vi "FPGA_9505_Thruster_PWMGeneratorOnly_NoCurrentFBack.vi"() -> ()   [LabVIEW 2012]
uses:
  <vilib>/LabVIEW Targets/FPGA/cRIO/cRIO-9505/controls.llb/_nicrio_cRIO-9505_DriveStatus.ctl
  <vilib>/Platform/TimedLoop/XDataNode/timing_clust.ctl
  <vilib>/Platform/TimedLoop/XDataNode/nitl_modes.ctl
  <vilib>/Platform/TimedLoop/XDataNode/wakeup.ctl
  <vilib>/LabVIEW Targets/FPGA/cRIO/cRIO-9505/controls.llb/_nicrio_cRIO-9505_DriveDirection.ctl
  <vilib>/rvi/Emulation/niFpgaSctlEmulationRegisterWithScheduler.vi
  <vilib>/rvi/Emulation/niFpgaSctlEmulationScheduler.vi
  <vilib>/rvi/eio/common/nirviEmuTemplateMethod_errors.vi
  <vilib>/rvi/eio/common/nirviEmuTemplatePropertyGet_noerrors.vi
  <vilib>/rvi/Emulation/niFpgaSctlEmulationGlobalWrite.vi
  <vilib>/Platform/TimedLoop/XDataNode/XDataNode.xnode
  <vilib>/eio/EIONode/EIONode.xnode
  <vilib>/eio/EIOMethodNode/EIOMethodNode.xnode
  <vilib>/eio/EIOPropertyNode/EIOPropertyNode.xnode
  <vilib>/rvi/eio/common/nirviEmuTemplatePropertyGet_errors.vi
  <vilib>/rvi/eio/common/nirviEmuTemplatePropertySet_errors.vi
  <vilib>/rvi/eio/common/nirviEmuTemplatePropertySet_noerrors.vi
  <vilib>/Platform/TimedLoop/XDataNode/XDNodeRunTimeDep.lvlib
panel:
  in  "Tab Control":enum32{"Control", "Debugging 1", "Debugging 2"}(tab)
  out "PWM Duty Cycle 1":i16
  in  "Input PWM Loop\nRate (usec) 1":u32=50
  in  "Input PWM 1":i16 caption="Setpoint"
  out "PWM Duty Cycle 2":i16
  in  "Input PWM Loop\nRate (usec) 2":u32=50
  in  "Input PWM 2":i16 caption="Setpoint"
  out "PWM Loop Counter 1":i32(graph)
  out "Sample Current Loop Counter 1":i32(graph)
  out "Current Sense 1":i16(graph)
  in  "Trig AI 1":bool
  out "PWM Duty Cycle 1":i16(graph)
  out "Input PWM Loop Counter 1":i32(graph)
  out "PWM Loop Counter 2":i32(graph)
  out "PWM Duty Cycle 2":i16(graph)
  out "Input PWM Loop Counter 2":i32(graph)
  in  "Trig AI 2":bool
  out "Current Sense 2":i16(graph)
  out "Sample Current Loop Counter 2":i32(graph)
  out "Vsup Present 2":bool
  out "Drive Fault 2":bool
  out "Drive Status 2":T1
  out "Temp Fault 2":bool
  in  "Enable\nDrive 2":bool
  in  "Disable\nDrive 2":bool
  out "Vsup Present 1":bool
  out "Drive Fault 1":bool
  out "Drive Status 1":T1
  out "Temp Fault 1":bool
  in  "Enable\nDrive 1":bool
  in  "Disable\nDrive 1":bool
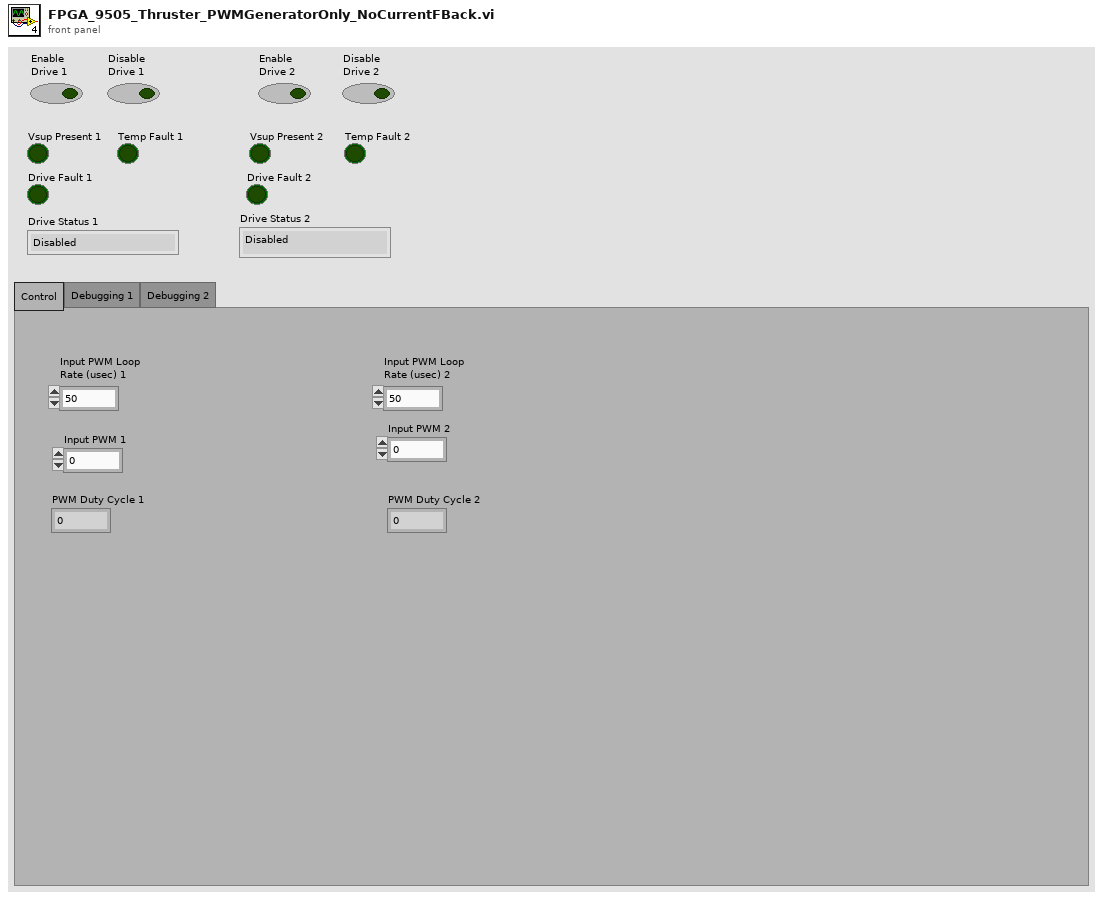
[diagram p1: front panel]
types:
  T1 = typedef "_nicrio_cRIO-9505_DriveStatus.ctl" = enum8{"Enabled", "Disabled", "Disabled by Drive Fault", "Disabled by Temp. Fault", "Disabled by E-Stop", "Unknown"}
  T2 = typedef "XDNodeRunTimeDep.lvlib/timing_clust.ctl" = cluster{"Expected End [f-1]":u64, "Actual End [f-1]":u64, "Finished Late? [f-1]":bool, "Expected End [i-1]":u64, "Actual End [i-1]":u64, "Finished Late? [i-1]":bool, "Expected Start [i]":u64, "Actual Start [i]":u64, "Expected Start [f]":u64, "Actual Start [f]":u64, "Source Name":string, "Structure Name":string, "Period":i64, "Deadline":i64, "Offset":i64, "Start":i64, "Priority":i32, "Timeout":i32, "Mode":T3, "Wakeup Reason":T4, "Error":errorcluster, "Source Type":string, "Secondary Source Type":string, "Global End Time":u64, "Global Start Time":u64, "Frame Duration":u64, "Iteration Duration":u64, "Assigned CPU":i32, "I/O Scan Engine Mode":u32}
  T3 = typedef "XDNodeRunTimeDep.lvlib/nitl_modes.ctl" = enum32{"No Change", "Process missed periods, maintain original phase", "Discard missed periods, maintain original phase", "Process missed periods, ignore original phase", "Discard missed periods, ignore original phase"}
  T4 = typedef "XDNodeRunTimeDep.lvlib/wakeup.ctl" = enum32{"Normal", "Aborted", "Asynchronous wakeup", "Timing source error", "Timed loop error", "Timeout"}
  T5 = typedef "_nicrio_cRIO-9505_DriveDirection.ctl" = enum8{"Clockwise", "Counterclockwise"}
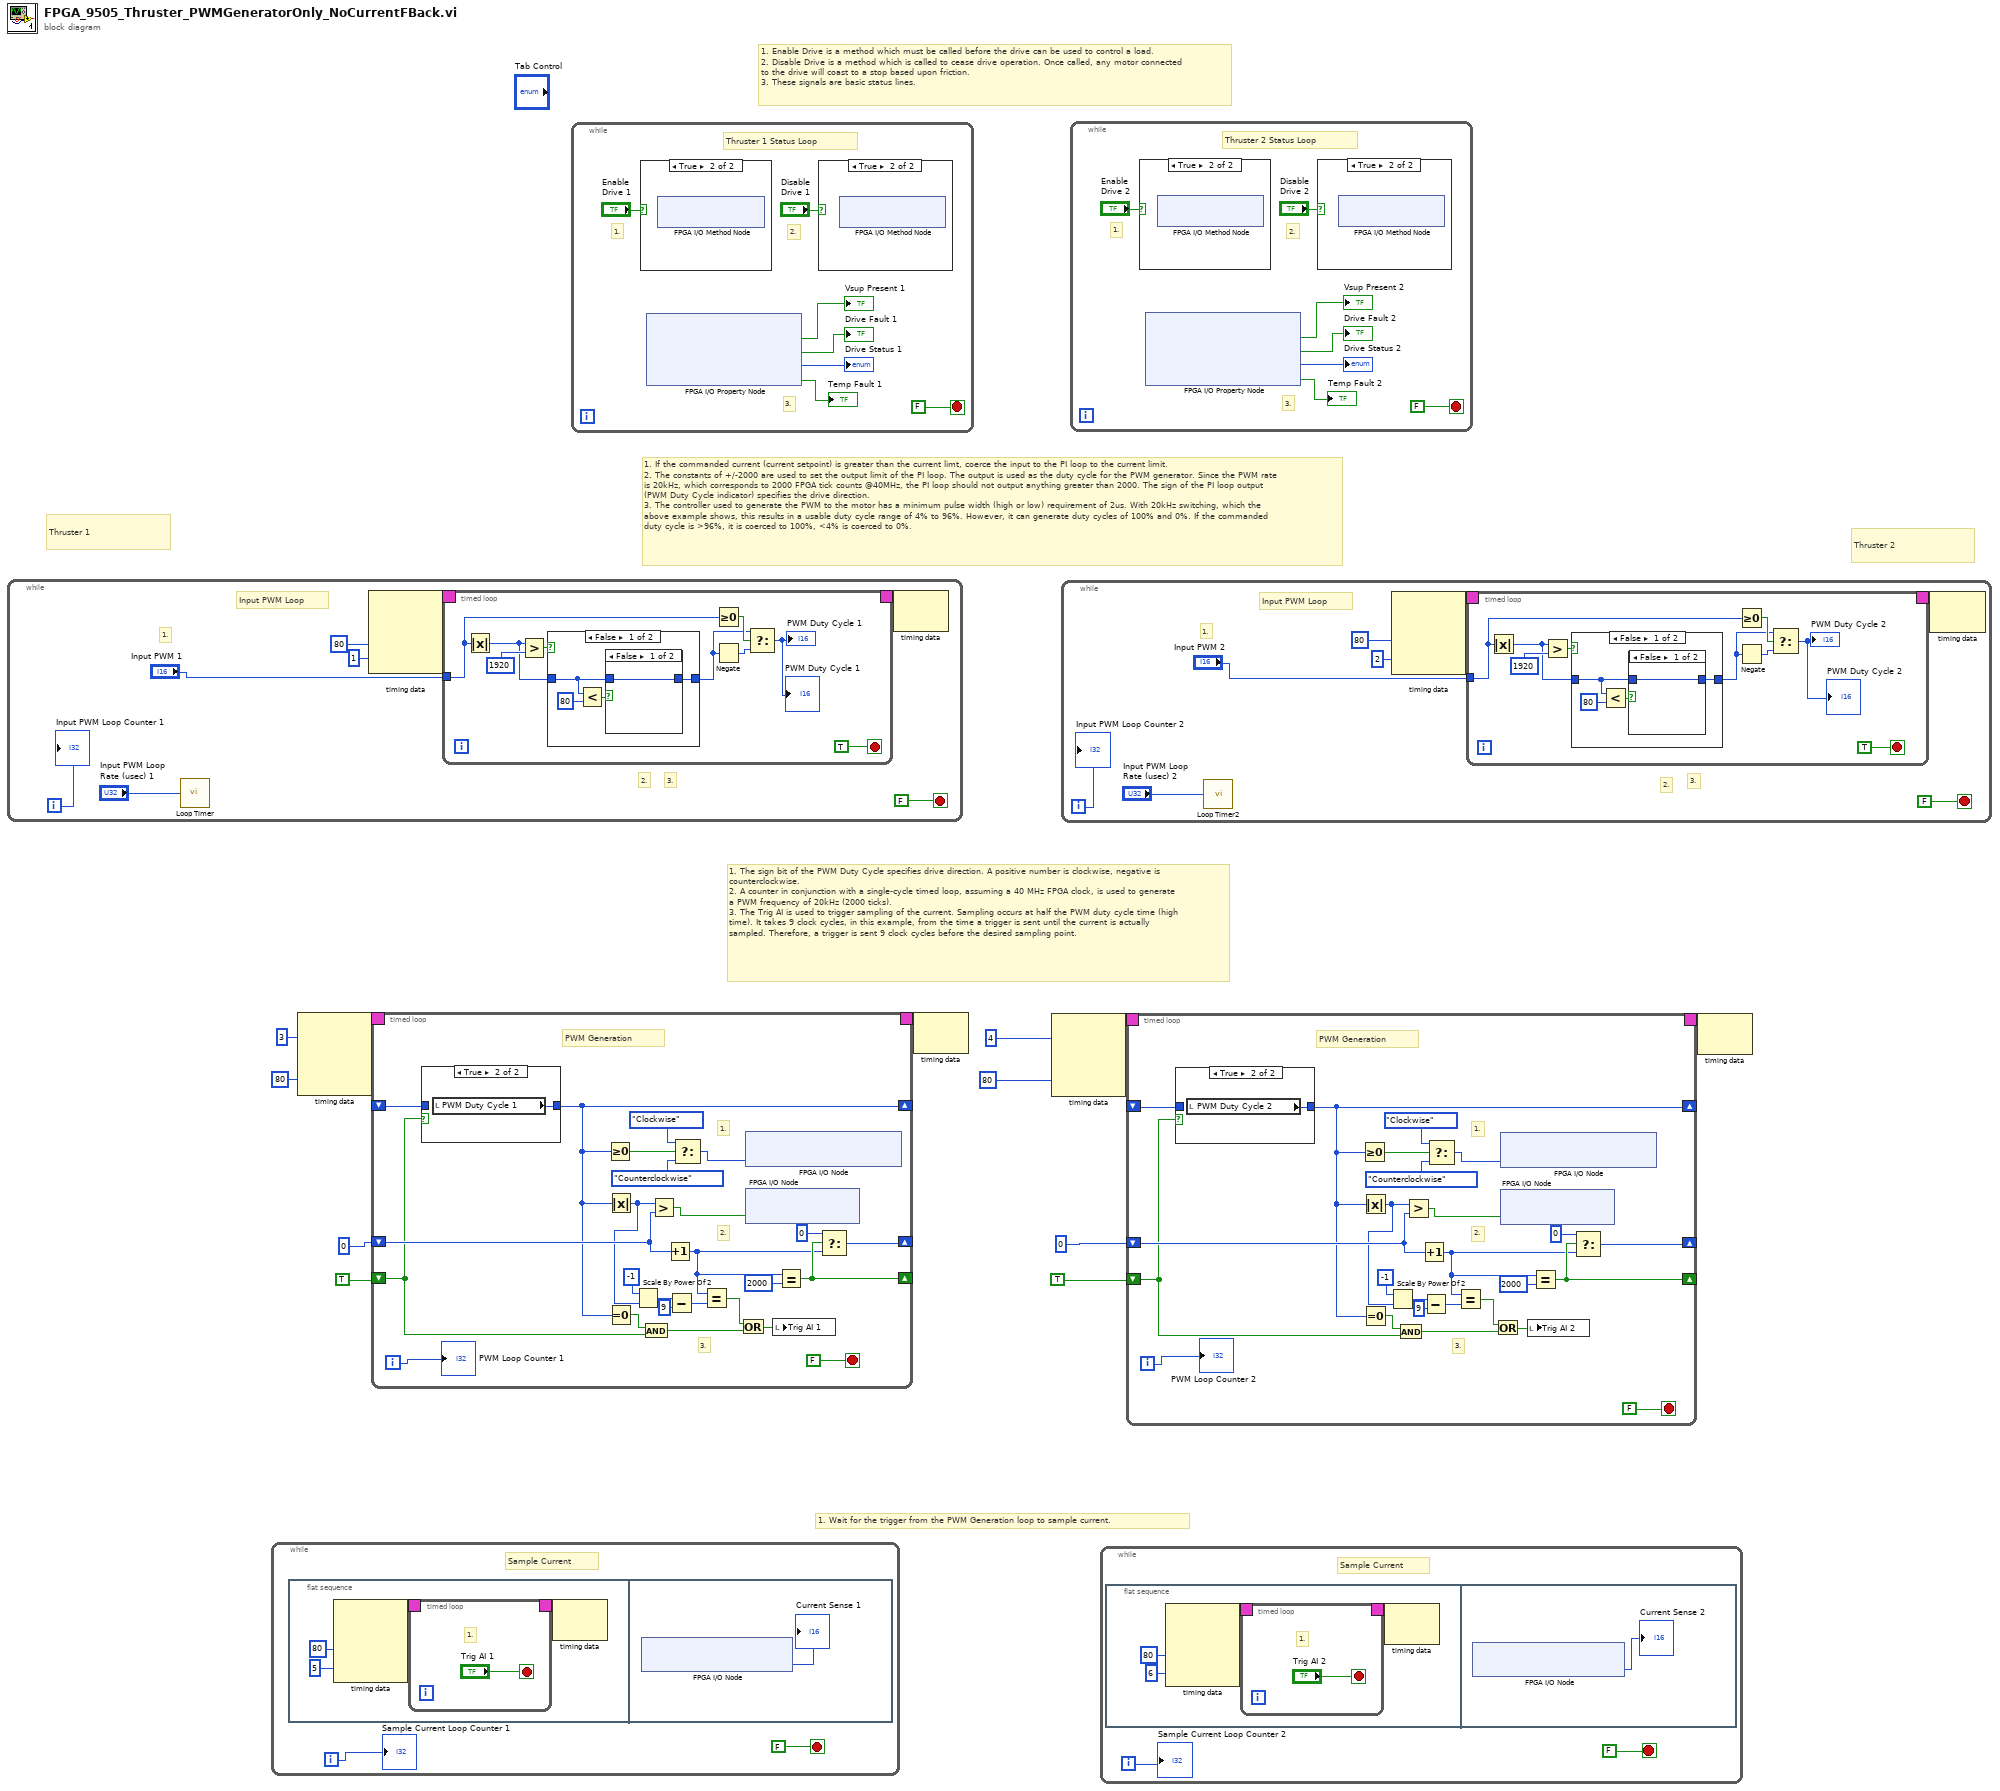
[diagram p0: block diagram]
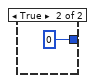
[diagram p4: hidden frame]
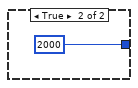
[diagram p5: hidden frame]
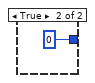
[diagram p6: hidden frame]
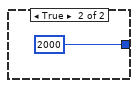
[diagram p7: hidden frame]
diagram:
  # "1. Wait for the trigger from the PWM Generation loop to sample current."
  # "1. The sign bit of the PWM Duty Cycle specifies drive direction. A positive number is clockwise, negative is counterclockwise.\n2. A counter in conjunction with a single-cycle timed loop, assuming a 40 MHz FPGA clock, is used to generate a PWM frequency of 20kHz (2000 ticks).\n3. The Trig AI is used to trigger sampling of the current. Sampling occurs at half the PWM duty cycle time (high time). It takes 9 clock cycles, in this example, from the time a trigger is sent until the current is actually sampled. Therefore, a trigger is sent 9 clock cycles before the desired sampling point."
  # "1. If the commanded current (current setpoint) is greater than the current limt, coerce the input to the PI loop to the current limit.\n2. The constants of +/-2000 are used to set the output limit of the PI loop. The output is used as the duty cycle for the PWM generator. Since the PWM rate is 20kHz, which corresponds to 2000 FPGA tick counts @40MHz, the PI loop should not output anything greater than 2000. The sign of the PI loop output (PWM Duty Cycle indicator) specifies the drive direction.\n3. The controller used to generate the PWM to the motor has a minimum pulse width (high or low) requirement of 2us. With 20kHz switching, which the above example shows, this results in a usable duty cycle range of 4% to 96%. However, it can generate duty cycles of 100% and 0%. If the commanded duty c..."
  # "Thruster 2"
  # "Thruster 1"
  # "1. Enable Drive is a method which must be called before the drive can be used to control a load.\n2. Disable Drive is a method which is called to cease drive operation. Once called, any motor connected to the drive will coast to a stop based upon friction.\n3. These signals are basic status lines."
  n1 = while {
    i -> [w16]
    stop <- FALSE stop-if-true
    # "2."
    # "3."
    # "1."
    # "Input PWM Loop"
    n2 = call "Loop Timer"("Count(uSec)"="Input PWM Loop\nRate (usec) 1") -> ()  [unwired: 1 out]
    n3 = node-c288(80, 1) -> (w19:T2)  [unwired: 2 out]
    n4 = timed-loop {
      timing: w19 -> [_]
      timing-out: [_] -> w18
      tunnel: "Input PWM 1" -> [w23]
      stop <- TRUE stop-if-true
      n5 = Absolute Value(x=w23) -> (abs(x)=w24:i16)
      n6 = Greater?(x=w24, y=i16 1920) -> (0:w26:bool)
      n7 = case shown="False" w26 {
        tunnel: [w32 i16 2000] -> w25
        tunnel: w24 -> [w30 _]
        frame False {
          n8 = Less?(x=w30, y=i16 80) -> (x < y?=w31:bool)
          n9 = case shown="False" w31 {
            tunnel: [w34 i16 0] -> w32
            tunnel: w30 -> [w34 _]
            frame False {
            }
            frame True {
            }
          }
        }
        frame True {
        }
      }
      n10 = Greater Or Equal To 0?(x=w23) -> (x >= 0?=w29:bool)
      n11 = Negate(x=w25) -> (-x=w28:i16)
      n12 = Select(t=w25, s=w29, f=w28) -> (s? t:f=→"PWM Duty Cycle 1" →"PWM Duty Cycle 1":i16)
    }
    n13 = node-c288(w18) -> ()  [unwired: 1 out]
    "Input PWM Loop Counter 1" <- w16
  }
  n14 = while {
    i -> [w44]
    stop <- FALSE stop-if-true
    # "Sample Current"
    n15 = flat-sequence {
      frame #0 {
        n16 = node-c288(80, 5) -> (w49:T2)  [unwired: 2 out]
        n17 = timed-loop {
          timing: w49 -> [_]
          timing-out: [_] -> w48
          stop <- "Trig AI 1" stop-if-true
          # "1."
        }
        n18 = node-c288(w48) -> ()  [unwired: 1 out]
      }
      frame #1 {
        n19 = xnode "FPGA I/O Node"() -> ("Mod2/Current Sense 2"=→"Current Sense 1":i16)  [unwired: 1 in, 1 out]
      }
    }
    "Sample Current Loop Counter 1" <- w44
  }
  n20 = node-c288(3, 80) -> (w12:T2)  [unwired: 2 in]
  n21 = timed-loop {
    timing: w12 -> [_]
    timing-out: [_] -> w11
    shift-right: [w80] -> _
    shift-left: i16 0 -> [w83]
    shift-right: [w79] -> _
    shift-left: TRUE -> [w76]
    shift-right: [w65] -> _
    shift-left: _ -> [w78]
    i -> [w59]
    stop <- FALSE stop-if-true
    # "3."
    # "2."
    # "1."
    # "PWM Generation"
    n22 = case shown="True" w76 {
      tunnel: [w84 w85] -> w65
      tunnel: w78 -> [w84 _]
      frame False {
      }
      frame True {
        n23 = local read "PWM Duty Cycle 1"() -> (w85:i16)
      }
    }
    n24 = Greater Or Equal To 0?(x=w65) -> (x >= 0?=w72:bool)
    n25 = Absolute Value(x=w65) -> (abs(x)=w63:i16)
    n26 = Equal To 0?(x=w65) -> (x = 0?=w77:bool)
    n27 = Scale By Power Of 2(n=i8 -1, x=w63) -> (x*2^n=w67:i16)
    n28 = And(x=w77, y=w76) -> (x .and. y?=w73:bool)
    n29 = Greater?(x=w63, y=w83) -> (0:w60:bool)
    n30 = Increment(x=w83) -> (x+1=w75:i16)
    n31 = Subtract(x=w67, y=i8 9) -> (x-y=w66:i16)
    n32 = Select(t=_nicrio_cRIO-9505_DriveDirection."Clockwise", s=w72, f=_nicrio_cRIO-9505_DriveDirection."Counterclockwise") -> (s? t:f=w61:T5)
    n33 = Equal?(x=w75, y=w66) -> (x = y?=w74:bool)
    n34 = Or(x=w74, y=w73) -> (x .or. y?=w69:bool)
    n35 = xnode "FPGA I/O Node"("Mod2/Drive Direction 2"=w61) -> ()  [unwired: 1 in, 1 out]
    n36 = xnode "FPGA I/O Node"("Mod2/Motor 2"=w60) -> ()  [unwired: 1 in, 1 out]
    n37 = local write "Trig AI 1"(w69) -> ()
    n38 = Equal?(x=w75, y=i16 2000) -> (x = y?=w79:bool)
    n39 = Select(t=i16 0, s=w79, f=w75) -> (s? t:f=w80:i16)
    "PWM Loop Counter 1" <- w59
  }
  n40 = while {
    stop <- FALSE stop-if-true
    # "3."
    # "2."
    # "1."
    # "Thruster 1 Status Loop"
    n41 = case shown="True" "Enable\nDrive 1" {
      frame False {
      }
      frame True {
        n42 = xnode "FPGA I/O Method Node"() -> ()  [unwired: 1 in, 1 out]
      }
    }
    n43 = xnode "FPGA I/O Property Node"() -> ("Vsup Present"=→"Vsup Present 1":bool, "Drive Fault"=→"Drive Fault 1":bool, "Drive Status"=→"Drive Status 1":T1, "Over Temperature Fault"=→"Temp Fault 1":bool)  [unwired: 1 in, 1 out]
    n44 = case shown="True" "Disable\nDrive 1" {
      frame False {
      }
      frame True {
        n45 = xnode "FPGA I/O Method Node"() -> ()  [unwired: 1 in, 1 out]
      }
    }
  }
  n46 = node-c288(w11) -> ()  [unwired: 1 out]
  n47 = node-c288(4, 80) -> (w10:T2)  [unwired: 2 in]
  n48 = while {
    i -> [w98]
    stop <- FALSE stop-if-true
    # "3."
    # "2."
    # "1."
    # "Input PWM Loop"
    n49 = call "Loop Timer2"("Count(uSec)"="Input PWM Loop\nRate (usec) 2") -> ()  [unwired: 1 out]
    n50 = node-c288(80, 2) -> (w101:T2)  [unwired: 2 out]
    n51 = timed-loop {
      timing: w101 -> [_]
      timing-out: [_] -> w100
      tunnel: "Input PWM 2" -> [w105]
      stop <- TRUE stop-if-true
      n52 = Absolute Value(x=w105) -> (abs(x)=w106:i16)
      n53 = Greater?(x=w106, y=i16 1920) -> (0:w108:bool)
      n54 = case shown="False" w108 {
        tunnel: [w114 i16 2000] -> w107
        tunnel: w106 -> [w112 _]
        frame False {
          n55 = Less?(x=w112, y=i16 80) -> (x < y?=w113:bool)
          n56 = case shown="False" w113 {
            tunnel: [w116 i16 0] -> w114
            tunnel: w112 -> [w116 _]
            frame False {
            }
            frame True {
            }
          }
        }
        frame True {
        }
      }
      n57 = Greater Or Equal To 0?(x=w105) -> (x >= 0?=w111:bool)
      n58 = Negate(x=w107) -> (-x=w110:i16)
      n59 = Select(t=w107, s=w111, f=w110) -> (s? t:f=→"PWM Duty Cycle 2" →"PWM Duty Cycle 2":i16)
    }
    n60 = node-c288(w100) -> ()  [unwired: 1 out]
    "Input PWM Loop Counter 2" <- w98
  }
  n61 = while {
    stop <- FALSE stop-if-true
    # "3."
    # "2."
    # "1."
    # "Thruster 2 Status Loop"
    n62 = case shown="True" "Enable\nDrive 2" {
      frame False {
      }
      frame True {
        n63 = xnode "FPGA I/O Method Node"() -> ()  [unwired: 1 in, 1 out]
      }
    }
    n64 = xnode "FPGA I/O Property Node"() -> ("Vsup Present"=→"Vsup Present 2":bool, "Drive Fault"=→"Drive Fault 2":bool, "Drive Status"=→"Drive Status 2":T1, "Over Temperature Fault"=→"Temp Fault 2":bool)  [unwired: 1 in, 1 out]
    n65 = case shown="True" "Disable\nDrive 2" {
      frame False {
      }
      frame True {
        n66 = xnode "FPGA I/O Method Node"() -> ()  [unwired: 1 in, 1 out]
      }
    }
  }
  n67 = while {
    i -> [w133]
    stop <- FALSE stop-if-true
    # "Sample Current"
    n68 = flat-sequence {
      frame #0 {
        n69 = node-c288(80, 6) -> (w138:T2)  [unwired: 2 out]
        n70 = timed-loop {
          timing: w138 -> [_]
          timing-out: [_] -> w137
          stop <- "Trig AI 2" stop-if-true
          # "1."
        }
        n71 = node-c288(w137) -> ()  [unwired: 1 out]
      }
      frame #1 {
        n72 = xnode "FPGA I/O Node"() -> ("Mod4/Current Sense 2"=→"Current Sense 2":i16)  [unwired: 1 in, 1 out]
      }
    }
    "Sample Current Loop Counter 2" <- w133
  }
  n73 = timed-loop {
    timing: w10 -> [_]
    timing-out: [_] -> w9
    shift-right: [w169] -> _
    shift-left: i16 0 -> [w172]
    shift-right: [w168] -> _
    shift-left: TRUE -> [w165]
    shift-right: [w154] -> _
    shift-left: _ -> [w167]
    i -> [w148]
    stop <- FALSE stop-if-true
    # "3."
    # "2."
    # "1."
    # "PWM Generation"
    n74 = case shown="True" w165 {
      tunnel: [w173 w174] -> w154
      tunnel: w167 -> [w173 _]
      frame False {
      }
      frame True {
        n75 = local read "PWM Duty Cycle 2"() -> (w174:i16)
      }
    }
    n76 = Greater Or Equal To 0?(x=w154) -> (x >= 0?=w161:bool)
    n77 = Absolute Value(x=w154) -> (abs(x)=w152:i16)
    n78 = Equal To 0?(x=w154) -> (x = 0?=w166:bool)
    n79 = Scale By Power Of 2(n=i8 -1, x=w152) -> (x*2^n=w156:i16)
    n80 = And(x=w166, y=w165) -> (x .and. y?=w162:bool)
    n81 = Greater?(x=w152, y=w172) -> (0:w149:bool)
    n82 = Increment(x=w172) -> (x+1=w164:i16)
    n83 = Subtract(x=w156, y=i8 9) -> (x-y=w155:i16)
    n84 = Select(t=_nicrio_cRIO-9505_DriveDirection."Clockwise", s=w161, f=_nicrio_cRIO-9505_DriveDirection."Counterclockwise") -> (s? t:f=w150:T5)
    n85 = Equal?(x=w164, y=w155) -> (x = y?=w163:bool)
    n86 = Or(x=w163, y=w162) -> (x .or. y?=w158:bool)
    n87 = xnode "FPGA I/O Node"("Mod4/Drive Direction 2"=w150) -> ()  [unwired: 1 in, 1 out]
    n88 = xnode "FPGA I/O Node"("Mod4/Motor 2"=w149) -> ()  [unwired: 1 in, 1 out]
    n89 = local write "Trig AI 2"(w158) -> ()
    n90 = Equal?(x=w164, y=i16 2000) -> (x = y?=w168:bool)
    n91 = Select(t=i16 0, s=w168, f=w164) -> (s? t:f=w169:i16)
    "PWM Loop Counter 2" <- w148
  }
  n92 = node-c288(w9) -> ()  [unwired: 1 out]
